vi "WPI_DriverStationGet Robot Mode.vi"(10 "Finish":bool, 11 "DS Occurrence":refnum<k4>) -> (0 "Match Info out":T4={"Autonomous Elapsed Seconds"=0.0, "TeleOp Elapsed Seconds"=0.0, "Disabled Elapsed Seconds"=0.0, "Visited Autonomous"=FALSE, "Visited TeleOp"=FALSE, "Visited Disabled"=FALSE, "Autonomous Settings"={"Autonomous Style"=enum."Independent", "VI Refnum"=refnum}}, 1 "Control Word":T1, 2 "Call Context":T3, 3 "Robot Mode":T2)   [LabVIEW 2017]
doc: "This VI waits for control packets to arrive and determines what robot code to execute next, teletop, disable, etc. It also contains a state machine to give a first and last call context parameter and execution timings to robot code.\n\nThis software is licensed. Open the labview\\readme\\WPI Robotics Library Open Source License.txt file for more information."
uses:
  <vilib>/Rock Robotics/WPI/DriverStation/WPI_DriverStationMatch Info.ctl
  <vilib>/Rock Robotics/WPI/DriverStation/WPI_DriverStationDerivedRobotMode.ctl
  <vilib>/Rock Robotics/WPI/DriverStation/WPI_DriverStationRobotMode2.ctl
  <vilib>/Rock Robotics/SystemInterfaces/NetworkCommunication/NetComm_ControlWord.ctl
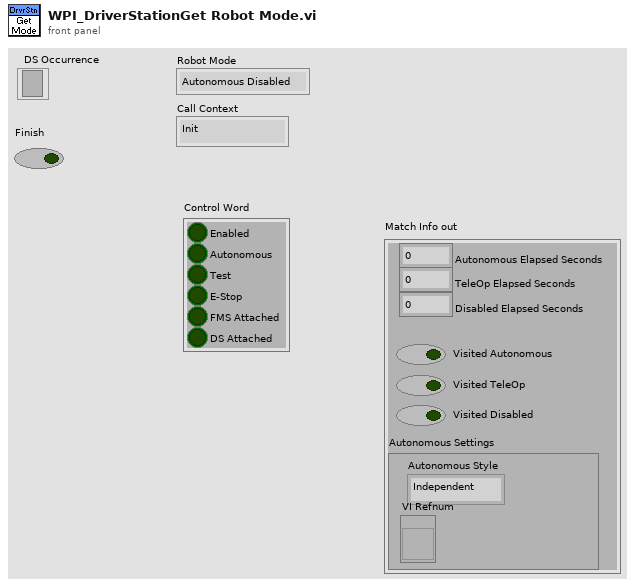
[diagram p1: front panel]
types:
  T1 = typedef "NetComm_ControlWord.ctl" = cluster{"Enabled":bool, "Autonomous":bool, "Test":bool, "E-Stop":bool, "FMS Attached":bool, "DS Attached":bool}
  T2 = typedef "WPI_DriverStationRobotMode2.ctl" = enum16{"Autonomous Disabled", "Autonomous Enabled", "Teleop Disabled", "Teleop Enabled", "Disconnected", "Finish", "Test Disabled", "Test Enabled", "Emergency Stopped"}
  T3 = typedef "WPI_DriverStationDerivedRobotMode.ctl" = enum16{"Init", "Execute", "Stop"}
  T4 = typedef "WPI_DriverStationMatch Info.ctl" = cluster{"Autonomous Elapsed Seconds":dbl, "TeleOp Elapsed Seconds":dbl, "Disabled Elapsed Seconds":dbl, "Visited Autonomous":bool, "Visited TeleOp":bool, "Visited Disabled":bool, "Autonomous Settings":cluster{"Autonomous Style":enum16{"Iterative", "Independent"}, "VI Refnum":refnum<vi>}}
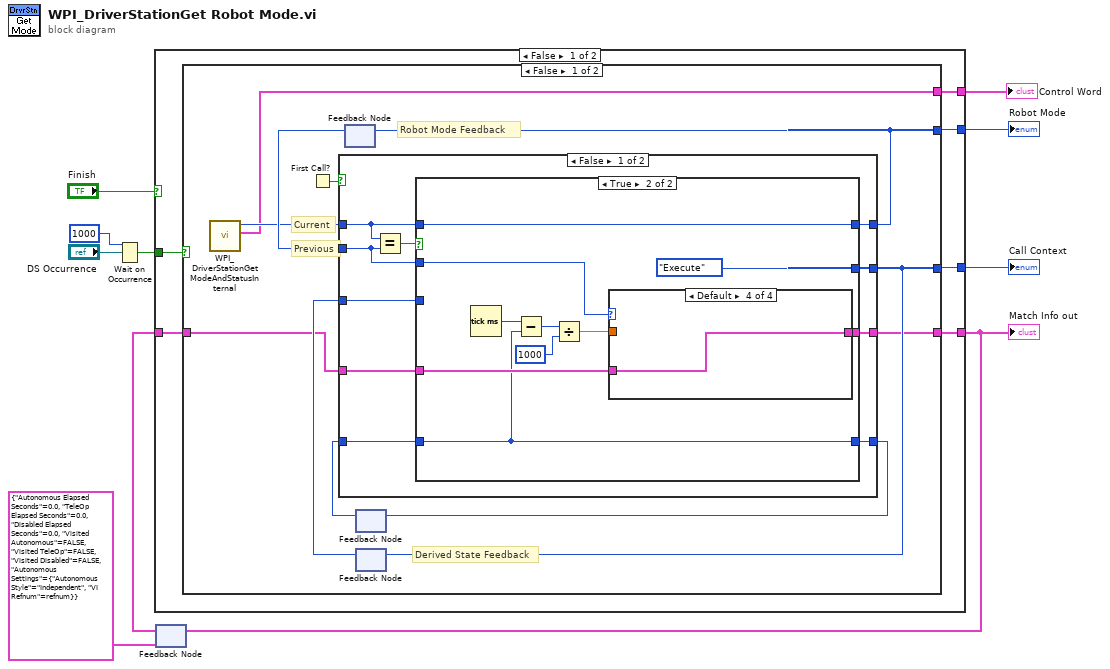
[diagram p0: block diagram]
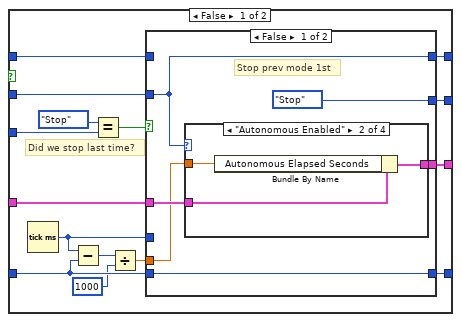
[diagram p2: hidden frame]
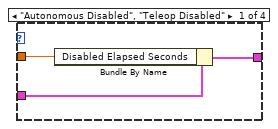
[diagram p3: hidden frame]
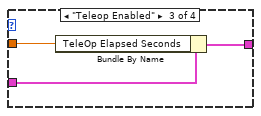
[diagram p4: hidden frame]
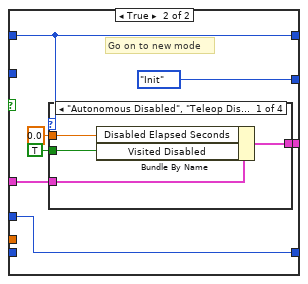
[diagram p6: hidden frame]
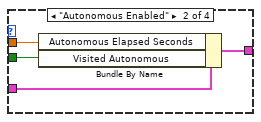
[diagram p7: hidden frame]
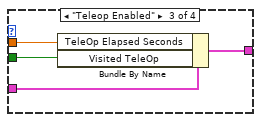
[diagram p8: hidden frame]
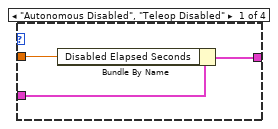
[diagram p10: hidden frame]
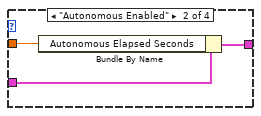
[diagram p11: hidden frame]
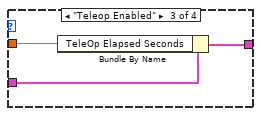
[diagram p12: hidden frame]
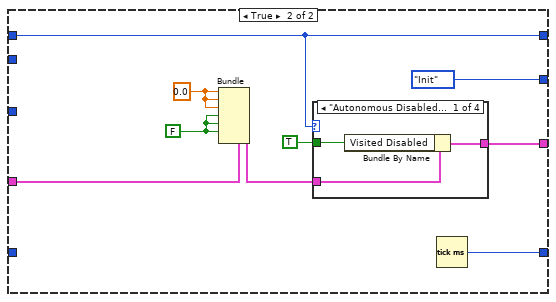
[diagram p13: hidden frame]
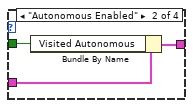
[diagram p14: hidden frame]
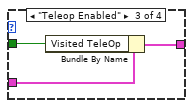
[diagram p15: hidden frame]
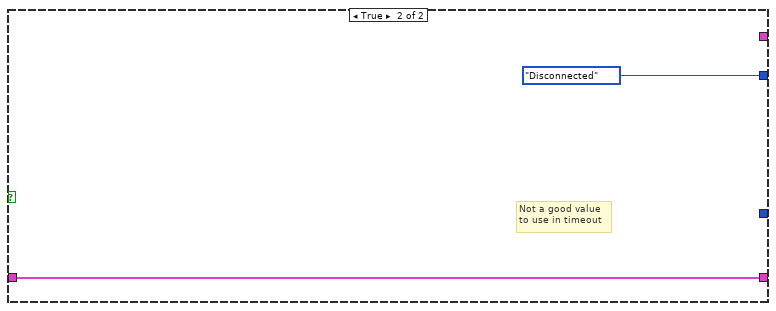
[diagram p17: hidden frame]
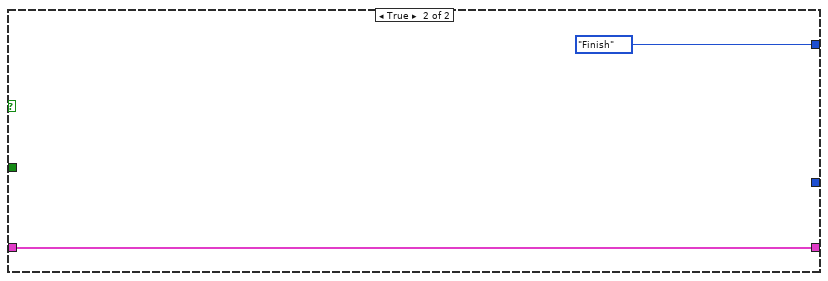
[diagram p18: hidden frame]
diagram:
  n1 = Wait on Occurrence(2:"DS Occurrence", 3:1000 ("ms timeout (-1)")) -> (0:w5:bool)  [unwired: 1 out]
  n2 = feedback #1(T4 {"Autonomous Elapsed Seconds"=0.0, "TeleOp Elapsed Seconds"=0.0, "Disabled Elapsed Seconds"=0.0, "Visited Autonomous"=FALSE, "Visited TeleOp"=FALSE, "Visited Disabled"=FALSE, "Autonomous Settings"={"Autonomous Style"=enum."Independent", "VI Refnum"=refnum}} ("Match Info")) -> (w9:T4)
  n3 = case shown="False" "Finish" {
    tunnel: [w16 _] -> w2
    tunnel: [w15 WPI_DriverStationRobotMode2."Finish" ("RobotMode")] -> w3
    tunnel: w5 -> [w14 _]
    tunnel: w9 -> [w13 w130]
    tunnel: [w12 w130] -> w8
    tunnel: [w11 _] -> w1
    frame False {
      n4 = case shown="False" w14 {
        tunnel: [w24 _] -> w16
        tunnel: [w23 WPI_DriverStationRobotMode2."Disconnected" ("RobotMode")] -> w15
        tunnel: w13 -> [w19 w128]
        tunnel: [w20 w128] -> w12
        tunnel: [w17 _] -> w11
        frame False {
          # "Derived State Feedback"
          # "Robot Mode Feedback"
          # "Previous"
          # "Current"
          n5 = call <vilib>:"WPI_DriverStationGetModeAndStatusInternal.vi"() -> ("Control Word"=w17:T1, "Robot Mode"=w18:T2)  [unwired: 10 in]
          n6 = First Call?() -> (First Call?: T/F=w25:bool)
          n7 = feedback #2() -> (w26:T2)  [unwired: 1 out]
          n8 = feedback #3() -> (w21:u32)  [unwired: 1 out]
          n9 = feedback #4() -> (w27:T3)  [unwired: 1 out]
          n10 = case shown="False" w25 {
            tunnel: [w37 w109] -> w23
            tunnel: [w36 WPI_DriverStationDerivedRobotMode."Init" ("Derived Robot State")] -> w24
            tunnel: w27 -> [w34 _]
            tunnel: w18 -> [w33 w109]
            tunnel: w26 -> [w32 _]
            tunnel: w19 -> [w31 w116]
            tunnel: [w30 w111] -> w20
            tunnel: [w28 w113] -> w22
            tunnel: w21 -> [w29 _]
            frame False {
              n11 = Equal?(x=w33, y=w32) -> (x = y?=w35:bool)
              n12 = case shown="True" w35 {
                tunnel: w33 -> [w50 w98]
                tunnel: [w49 w98] -> w37
                tunnel: [w48 WPI_DriverStationDerivedRobotMode."Execute" ("Derived Robot State")] -> w36
                tunnel: w34 -> [w52 _]
                tunnel: w32 -> [w47 w93]
                tunnel: w31 -> [w41 w94]
                tunnel: [w45 w95] -> w30
                tunnel: w29 -> [w42 w92]
                tunnel: [w43 w92] -> w28
                frame False {
                  # "Did we stop last time?"
                  n13 = Tick Count (ms)() -> (millisecond timer value=w44:u32)
                  n14 = Subtract(x=w44, y=w42) -> (x-y=w40:u32)
                  n15 = Equal?(x=WPI_DriverStationDerivedRobotMode."Stop" ("Derived Robot State"), y=w52) -> (x = y?=w51:bool)
                  n16 = Divide(x=w40, y=1000) -> (x/y=w39:dbl)
                  n17 = case shown="False" w51 {
                    tunnel: w50 -> [_ w74]
                    tunnel: [w53 w74] -> w49
                    tunnel: [WPI_DriverStationDerivedRobotMode."Stop" ("Derived Robot State") WPI_DriverStationDerivedRobotMode."Init" ("Derived Robot State")] -> w48
                    tunnel: w47 -> [w53 _]
                    tunnel: w41 -> [w56 w72]
                    tunnel: [w57 w71] -> w45
                    tunnel: w39 -> [w55 _]
                    tunnel: w44 -> [_ w69]
                    tunnel: [w54 w69] -> w43
                    tunnel: w42 -> [w54 _]
                    frame False {
                      # "Stop prev mode 1st"
                      n18 = case shown="\"Autonomous Enabled\"" w53 {
                        tunnel: w55 -> [w61 w64 w67 _]
                        tunnel: w56 -> [w60 w63 w66 w68]
                        tunnel: [w59 w62 w65 w68] -> w57
                        frame "Autonomous Disabled", "Teleop Disabled" {
                          n19 = Bundle By Name(cluster=w60, "Disabled Elapsed Seconds"=w61) -> (w59:T4)
                        }
                        frame "Autonomous Enabled" {
                          n20 = Bundle By Name(cluster=w63, "Autonomous Elapsed Seconds"=w64) -> (w62:T4)
                        }
                        frame "Teleop Enabled" {
                          n21 = Bundle By Name(cluster=w66, "TeleOp Elapsed Seconds"=w67) -> (w65:T4)
                        }
                        frame Default {
                        }
                      }
                    }
                    frame True {
                      # "Go on to new mode"
                      n22 = case shown="\"Autonomous Disabled\", \"Teleop Disabled\"" w74 {
                        tunnel: 0.0 -> [w79 w83 w84 _]
                        tunnel: w72 -> [w78 w82 w87 w88]
                        tunnel: [w77 w81 w86 w88] -> w71
                        tunnel: TRUE -> [w76 w80 w85 _]
                        frame "Autonomous Disabled", "Teleop Disabled" {
                          n23 = Bundle By Name(cluster=w78, "Disabled Elapsed Seconds"=w79, "Visited Disabled"=w76) -> (w77:T4)
                        }
                        frame "Autonomous Enabled" {
                          n24 = Bundle By Name(cluster=w82, "Autonomous Elapsed Seconds"=w83, "Visited Autonomous"=w80) -> (w81:T4)
                        }
                        frame "Teleop Enabled" {
                          n25 = Bundle By Name(cluster=w87, "TeleOp Elapsed Seconds"=w84, "Visited TeleOp"=w85) -> (w86:T4)
                        }
                        frame Default {
                        }
                      }
                    }
                  }
                }
                frame True {
                  n26 = Tick Count (ms)() -> (millisecond timer value=w96:u32)
                  n27 = Subtract(x=w96, y=w92) -> (x-y=w90:u32)
                  n28 = Divide(x=w90, y=u32 1000) -> (x/y=w91:dbl)
                  n29 = case shown="Default" w93 {
                    tunnel: w91 -> [w101 w104 w107 _]
                    tunnel: w94 -> [w100 w103 w106 w108]
                    tunnel: [w99 w102 w105 w108] -> w95
                    frame "Autonomous Disabled", "Teleop Disabled" {
                      n30 = Bundle By Name(cluster=w100, "Disabled Elapsed Seconds"=w101) -> (w99:T4)
                    }
                    frame "Autonomous Enabled" {
                      n31 = Bundle By Name(cluster=w103, "Autonomous Elapsed Seconds"=w104) -> (w102:T4)
                    }
                    frame "Teleop Enabled" {
                      n32 = Bundle By Name(cluster=w106, "TeleOp Elapsed Seconds"=w107) -> (w105:T4)
                    }
                    frame Default {
                    }
                  }
                }
              }
            }
            frame True {
              w115 = 0.0
              w114 = FALSE
              n33 = Bundle(cluster=w116, "Autonomous Elapsed Seconds"=w115, "TeleOp Elapsed Seconds"=w115, "Disabled Elapsed Seconds"=w115, "Visited Autonomous"=w114, "Visited TeleOp"=w114, "Visited Disabled"=w114) -> (w112:T4)  [unwired: 1 out]
              n34 = case shown="\"Autonomous Disabled\", \"Teleop Disabled\"" w109 {
                tunnel: w112 -> [w120 w123 w126 w127]
                tunnel: [w119 w122 w125 w127] -> w111
                tunnel: TRUE -> [w118 w121 w124 _]
                frame "Autonomous Disabled", "Teleop Disabled" {
                  n35 = Bundle By Name(cluster=w120, "Visited Disabled"=w118) -> (w119:T4)
                }
                frame "Autonomous Enabled" {
                  n36 = Bundle By Name(cluster=w123, "Visited Autonomous"=w121) -> (w122:T4)
                }
                frame "Teleop Enabled" {
                  n37 = Bundle By Name(cluster=w126, "Visited TeleOp"=w124) -> (w125:T4)
                }
                frame Default {
                }
              }
              n38 = Tick Count (ms)() -> (millisecond timer value=w113:u32)
            }
          }
          n39 = feedback-in #2(w23) -> ()
          n40 = feedback-in #3(w22) -> ()
          n41 = feedback-in #4(w24) -> ()
        }
        frame True {
          # "Not a good value\nto use in timeout"
        }
      }
    }
    frame True {
    }
  }
  "Robot Mode" <- w3
  "Call Context" <- w2
  "Match Info out" <- w8
  "Control Word" <- w1
  n42 = feedback-in #1(w8) -> ()
